vi "Filter SRs.vi"(8 "error in (no error)":errorcluster, 9 "Filter Cluster":T1, 11 "list in":T2[](array[typedef]) {"Last Updated" format="%<%x>T"}) -> (0 "error out":errorcluster, 3 "list out":T2[](array[typedef]) {"Last Updated" format="%<%x>T"})   [LabVIEW 2018]
uses:
  SR Cluster.ctl
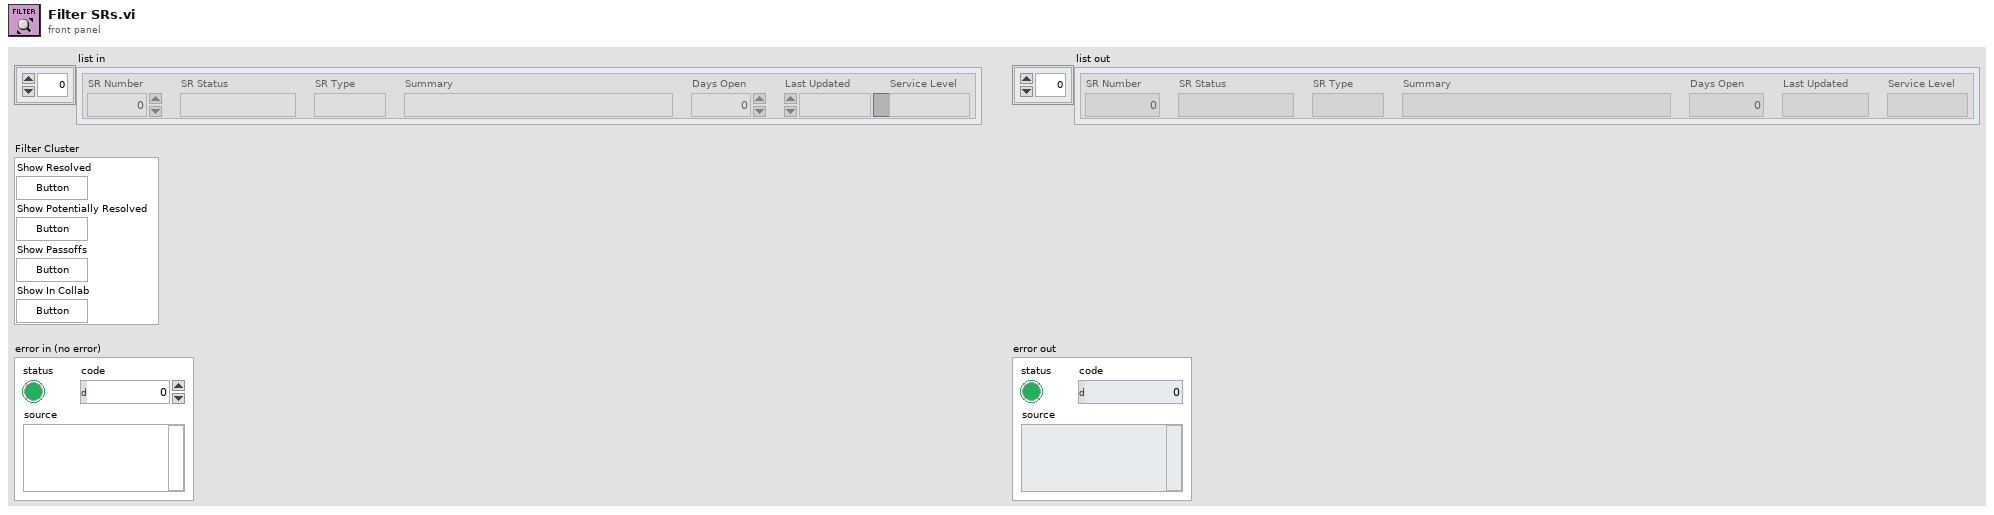
[diagram p1: front panel]
types:
  T1 = cluster{"Show Resolved":bool, "Show Potentially Resolved":bool, "Show Passoffs":bool, "Show In Collab":bool}
  T2 = typedef "SR Cluster.ctl" = cluster{"SR Number":i32, "SR Status":string, "SR Type":string, "Summary":string, "Days Open":dbl, "Last Updated":timestamp, "Service Level":string}
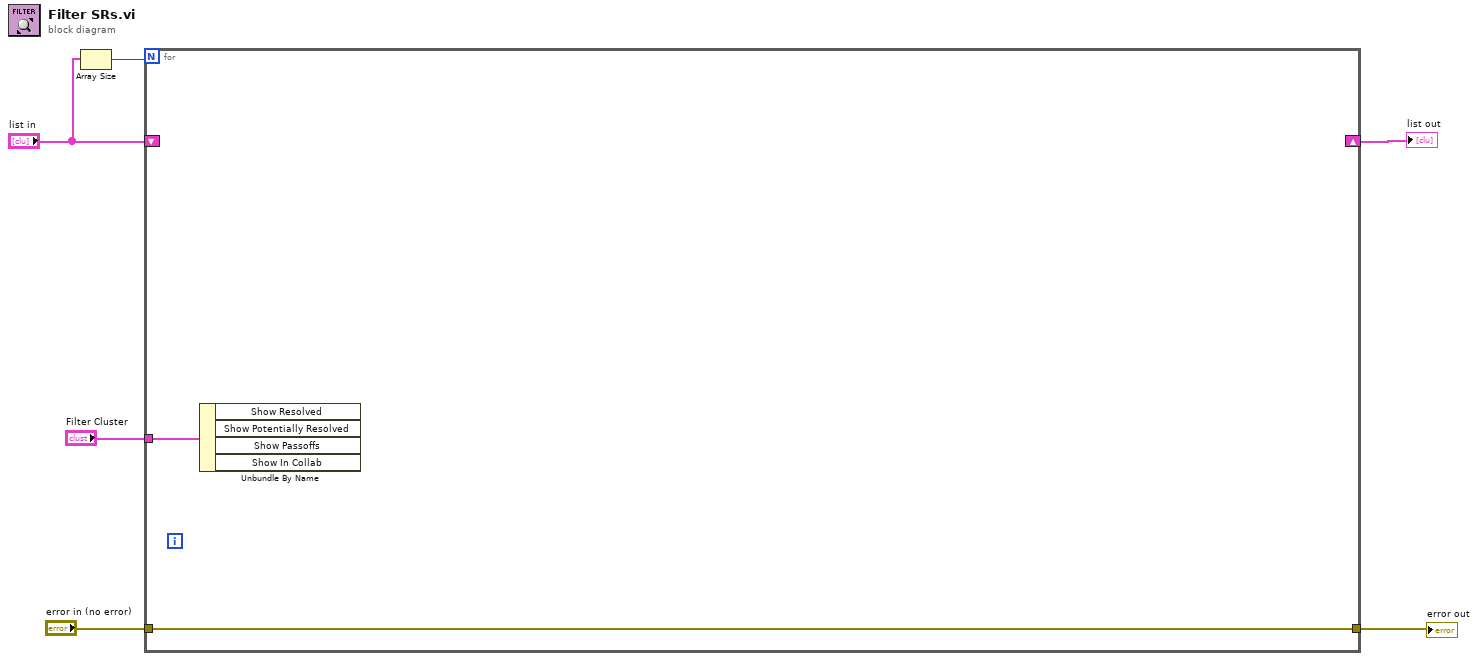
[diagram p0: block diagram]
diagram:
  n1 = Array Size(array="list in") -> (size(s)=w2:i32)
  n2 = for {
    N: w2 -> [_]
    tunnel: "Filter Cluster" -> [w7]
    tunnel: "error in (no error)" -> [w8]
    tunnel: [w8] -> w4
    shift-right: [_] -> w3
    shift-left: "list in" -> [_]
    n3 = Unbundle By Name(w7) -> ()  [unwired: 4 out]
  }
  "error out" <- w4
  "list out" <- w3
